vi "validate.vi"(8 "error in":errorcluster, 11 "Daqmx Module configuration in":refnum<class "DAQmx Module Configuration.lvclass">) -> (0 "error out":errorcluster, 3 "Daqmx Module configuration out":refnum<class "DAQmx Module Configuration.lvclass">)   [LabVIEW 2014, in "DAQmx Module Configuration.lvclass"]
doc: "This function performs validation of the configuration. This function should be safe to call at any point and should not rely on anything in the runtime environment."
uses:
  DAQmx Module Configuration.lvclass
  <vilib>/NI/Tag Bus Module Framework/module configuration/TBM module configuration.lvclass
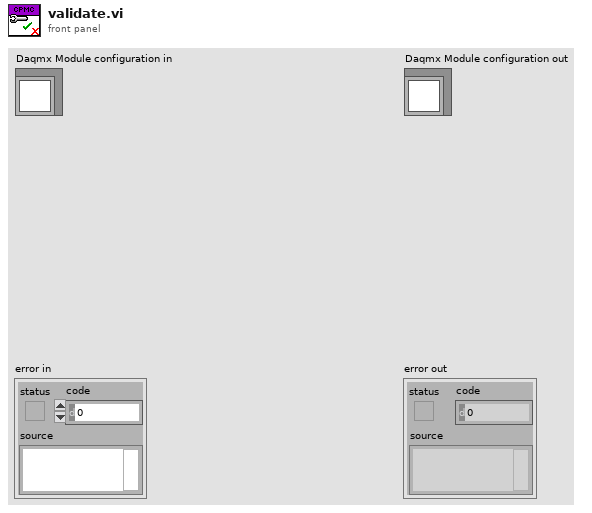
[diagram p1: front panel]
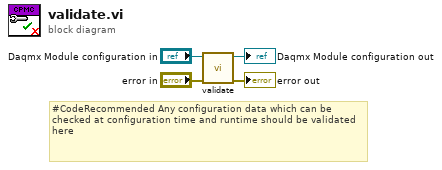
[diagram p0: block diagram]
diagram:
  # "#CodeRecommended Any configuration data which can be checked at configuration time and runtime should be validated here"
  n1 = call-parent "validate.vi"("error in"="error in", "configuration in"="Daqmx Module configuration in") -> ("error out"=→"error out":errorcluster, "configuration out"=→"Daqmx Module configuration out":refnum<class "DAQmx Module Configuration.lvclass">)  [unwired: 8 in]
